vi "Counter till 12.vi"() -> ()   [LabVIEW 2020]
panel:
  out "Buzzer":bool
  out "B":bool
  in  "clk":bool
  out "D":bool
  out "C":bool
  out "A":bool
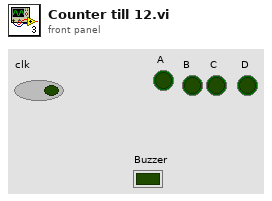
[diagram p1: front panel]
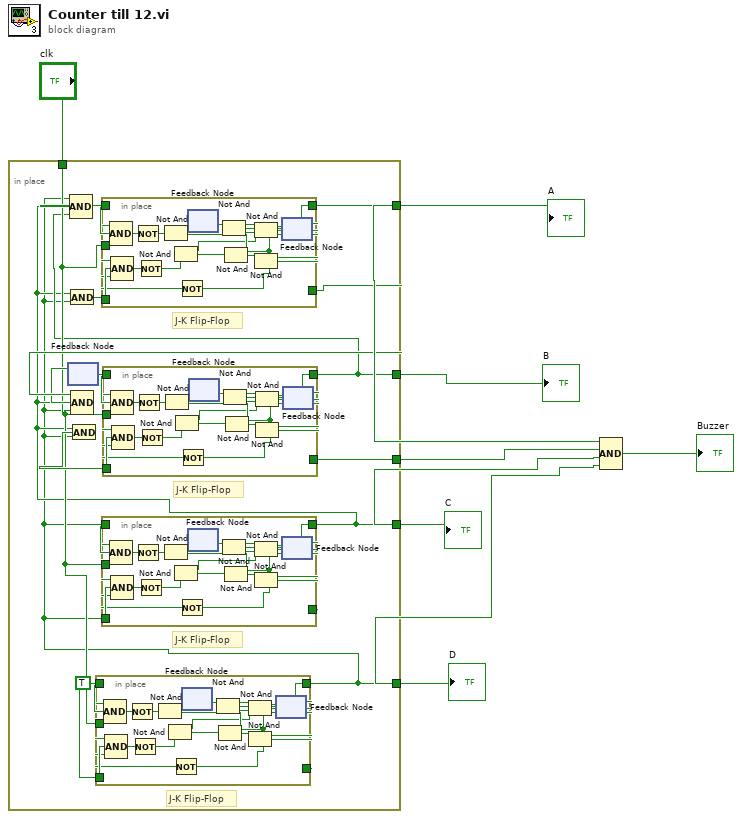
[diagram p0: block diagram]
diagram:
  n1 = in-place {
    in-place-border: "clk" -> [w13]
    in-place-border: [w12] -> w6
    in-place-border: [w11] -> w5
    in-place-border: [w10] -> w4
    in-place-border: [w9] -> w3
    in-place-border: [w8] -> w2
    w14 = TRUE
    # "J-K Flip-Flop"
    # "J-K Flip-Flop"
    # "J-K Flip-Flop"
    # "J-K Flip-Flop"
    n2 = feedback #1() -> (w16:bool)  [unwired: 1 in]
    n3 = in-place {
      in-place-border: w14 -> [w31]
      in-place-border: w14 -> [w30]
      in-place-border: w13 -> [w28]
      in-place-border: [w26] -> _
      in-place-border: [w25] -> w8
      n4 = Not(x=w28) -> (.not. x?=w29:bool)
      n5 = feedback #2() -> (w34:bool)  [unwired: 1 in]
      n6 = Not And(1:w29, 2:w34) -> (0:w33:bool)
      n7 = feedback #3() -> (w25:bool)  [unwired: 1 in]
      n8 = Compound Arithmetic op=AND(w28, w30, w25) -> (w22:bool)
      n9 = Not(x=w22) -> (.not. x?=w21:bool)
      n10 = Not And(1:w21, 2:w34) -> (0:w36:bool)
      n11 = Not And(1:w36, 2:w29) -> (0:w32:bool)
      n12 = Not And(1:w32, 2:w25) -> (0:w26:bool)
      n13 = Compound Arithmetic op=AND(w26, w31, w28) -> (w24:bool)
      n14 = Not(x=w24) -> (.not. x?=w23:bool)
      n15 = Not And(1:w36, 2:w23) -> (0:w35:bool)
      n16 = feedback-in #2(w35) -> ()
      n17 = Not And(1:w26, 2:w33) -> (0:w27:bool)
      n18 = feedback-in #3(w27) -> ()
    }
    n19 = in-place {
      in-place-border: w8 -> [w47]
      in-place-border: w8 -> [w46]
      in-place-border: w13 -> [w44]
      in-place-border: [w42] -> _
      in-place-border: [w41] -> w9
      n20 = Not(x=w44) -> (.not. x?=w45:bool)
      n21 = feedback #4() -> (w50:bool)  [unwired: 1 in]
      n22 = Not And(1:w45, 2:w50) -> (0:w49:bool)
      n23 = feedback #5() -> (w41:bool)  [unwired: 1 in]
      n24 = Compound Arithmetic op=AND(w44, w46, w41) -> (w38:bool)
      n25 = Not(x=w38) -> (.not. x?=w37:bool)
      n26 = Not And(1:w37, 2:w50) -> (0:w52:bool)
      n27 = Not And(1:w52, 2:w45) -> (0:w48:bool)
      n28 = Not And(1:w48, 2:w41) -> (0:w42:bool)
      n29 = Compound Arithmetic op=AND(w42, w47, w44) -> (w40:bool)
      n30 = Not(x=w40) -> (.not. x?=w39:bool)
      n31 = Not And(1:w52, 2:w39) -> (0:w51:bool)
      n32 = feedback-in #4(w51) -> ()
      n33 = Not And(1:w42, 2:w49) -> (0:w43:bool)
      n34 = feedback-in #5(w43) -> ()
    }
    n35 = And(x=w9, y=w8) -> (x .and. y?=w19:bool)
    n36 = And(x=w9, y=w8) -> (x .and. y?=w15:bool)
    n37 = in-place {
      in-place-border: w16 -> [w63]
      in-place-border: w15 -> [w62]
      in-place-border: w13 -> [w60]
      in-place-border: [w58] -> w10
      in-place-border: [w57] -> w12
      n38 = Not(x=w60) -> (.not. x?=w61:bool)
      n39 = feedback #6() -> (w66:bool)  [unwired: 1 in]
      n40 = Not And(1:w61, 2:w66) -> (0:w65:bool)
      n41 = feedback #7() -> (w57:bool)  [unwired: 1 in]
      n42 = Compound Arithmetic op=AND(w60, w62, w57) -> (w54:bool)
      n43 = Not(x=w54) -> (.not. x?=w53:bool)
      n44 = Not And(1:w53, 2:w66) -> (0:w68:bool)
      n45 = Not And(1:w68, 2:w61) -> (0:w64:bool)
      n46 = Not And(1:w64, 2:w57) -> (0:w58:bool)
      n47 = Compound Arithmetic op=AND(w58, w63, w60) -> (w56:bool)
      n48 = Not(x=w56) -> (.not. x?=w55:bool)
      n49 = Not And(1:w68, 2:w55) -> (0:w67:bool)
      n50 = feedback-in #6(w67) -> ()
      n51 = Not And(1:w58, 2:w65) -> (0:w59:bool)
      n52 = feedback-in #7(w59) -> ()
    }
    n53 = Compound Arithmetic op=AND(w8, w9, w12) -> (w20:bool)
    n54 = in-place {
      in-place-border: w20 -> [w79]
      in-place-border: w19 -> [w78]
      in-place-border: w13 -> [w76]
      in-place-border: [w74] -> w18
      in-place-border: [w73] -> w11
      n55 = Not(x=w76) -> (.not. x?=w77:bool)
      n56 = feedback #8() -> (w82:bool)  [unwired: 1 in]
      n57 = Not And(1:w77, 2:w82) -> (0:w81:bool)
      n58 = feedback #9() -> (w73:bool)  [unwired: 1 in]
      n59 = Compound Arithmetic op=AND(w76, w78, w73) -> (w70:bool)
      n60 = Not(x=w70) -> (.not. x?=w69:bool)
      n61 = Not And(1:w69, 2:w82) -> (0:w84:bool)
      n62 = Not And(1:w84, 2:w77) -> (0:w80:bool)
      n63 = Not And(1:w80, 2:w73) -> (0:w74:bool)
      n64 = Compound Arithmetic op=AND(w74, w79, w76) -> (w72:bool)
      n65 = Not(x=w72) -> (.not. x?=w71:bool)
      n66 = Not And(1:w84, 2:w71) -> (0:w83:bool)
      n67 = feedback-in #8(w83) -> ()
      n68 = Not And(1:w74, 2:w81) -> (0:w75:bool)
      n69 = feedback-in #9(w75) -> ()
    }
    n70 = Compound Arithmetic op=AND(w18, w9, w8) -> (w17:bool)
    n71 = feedback-in #1(w17) -> ()
  }
  "A" <- w5
  "C" <- w3
  "D" <- w2
  "B" <- w6
  n72 = Compound Arithmetic op=AND(w5, w4, w3, w2) -> (→"Buzzer":bool)
